vi "Test bearbeiten.vi"(6 "error in (no error)":errorcluster, 8 "Test in":refnum<class "Test.lvclass">, 9 "Data":T1={"Report.lvclass"=refnum, "Norm"="", "last State"=enum."Initialize", "Norm ID"=0, "parameter"=[], "EMTestCWS500N.lvclass"=refnum, "CEG4500.lvclass"=refnum, "Tektronix RSA5106A.lvclass"=refnum, "erfolgreich"=FALSE, "log"="", "Kommentar"="", "Device Enum"=enum."emTestCWS500N", "Test Enum"=enum."HF-Felder", "debug"=FALSE, "tab"=enum."Hauptmenü", "ESD Pistol.lvclass"=refnum, "SubPnl Refnum"=refnum, "TabCtl Refnum"=refnum, "ButtonsEinblenden?"=FALSE, "VKey"=enum."ASCII"}) -> (0 "error out":errorcluster, 1 "abbrechen":bool, 2 "Test out":refnum<class "Test.lvclass">)   [LabVIEW 2013, in "DataCreation.lvlib"]
uses:
  lib/DataCreation.lvlib
  Main/controls/Data.ctl
  classes/Datastructure/Report/Report.lvclass
  classes/Devices/emTestCWS500N/EMTestCWS500N.lvclass
  classes/Devices/CEG4500/CEG4500.lvclass
  classes/Devices/Tektronix RSA5106A/Tektronix RSA5106A.lvclass
  ESD Pistol.lvclass
  Main/controls/State.ctl
  classes/Devices/DeviceInterface/Devices.ctl
  classes/Tests/TestInterface/Tests.ctl
  Tabs.ctl
  <vilib>/event_ctls.llb/eventvkey.ctl
  classes/Datastructure/Test/Test.lvclass
  classes/Datastructure/Image/img.lvclass
  classes/Datastructure/Norm/Norm.lvclass
  lib/TreeRepresentation.lvlib
panel:
  in  "number of pictures":i32
  in  "Tab Control":enum32{"Test", "Daten"}(tab)
  in  "Cancel Button":bool
  in  "Tree pics":string(tree)
  in  "OK Button":bool
  in  "Add picture":bool
  in  "Kommentar":string
  in  "Test Name":string
  in  "Parameter":string[][](table)
  in  "Tree Report":string(tree)
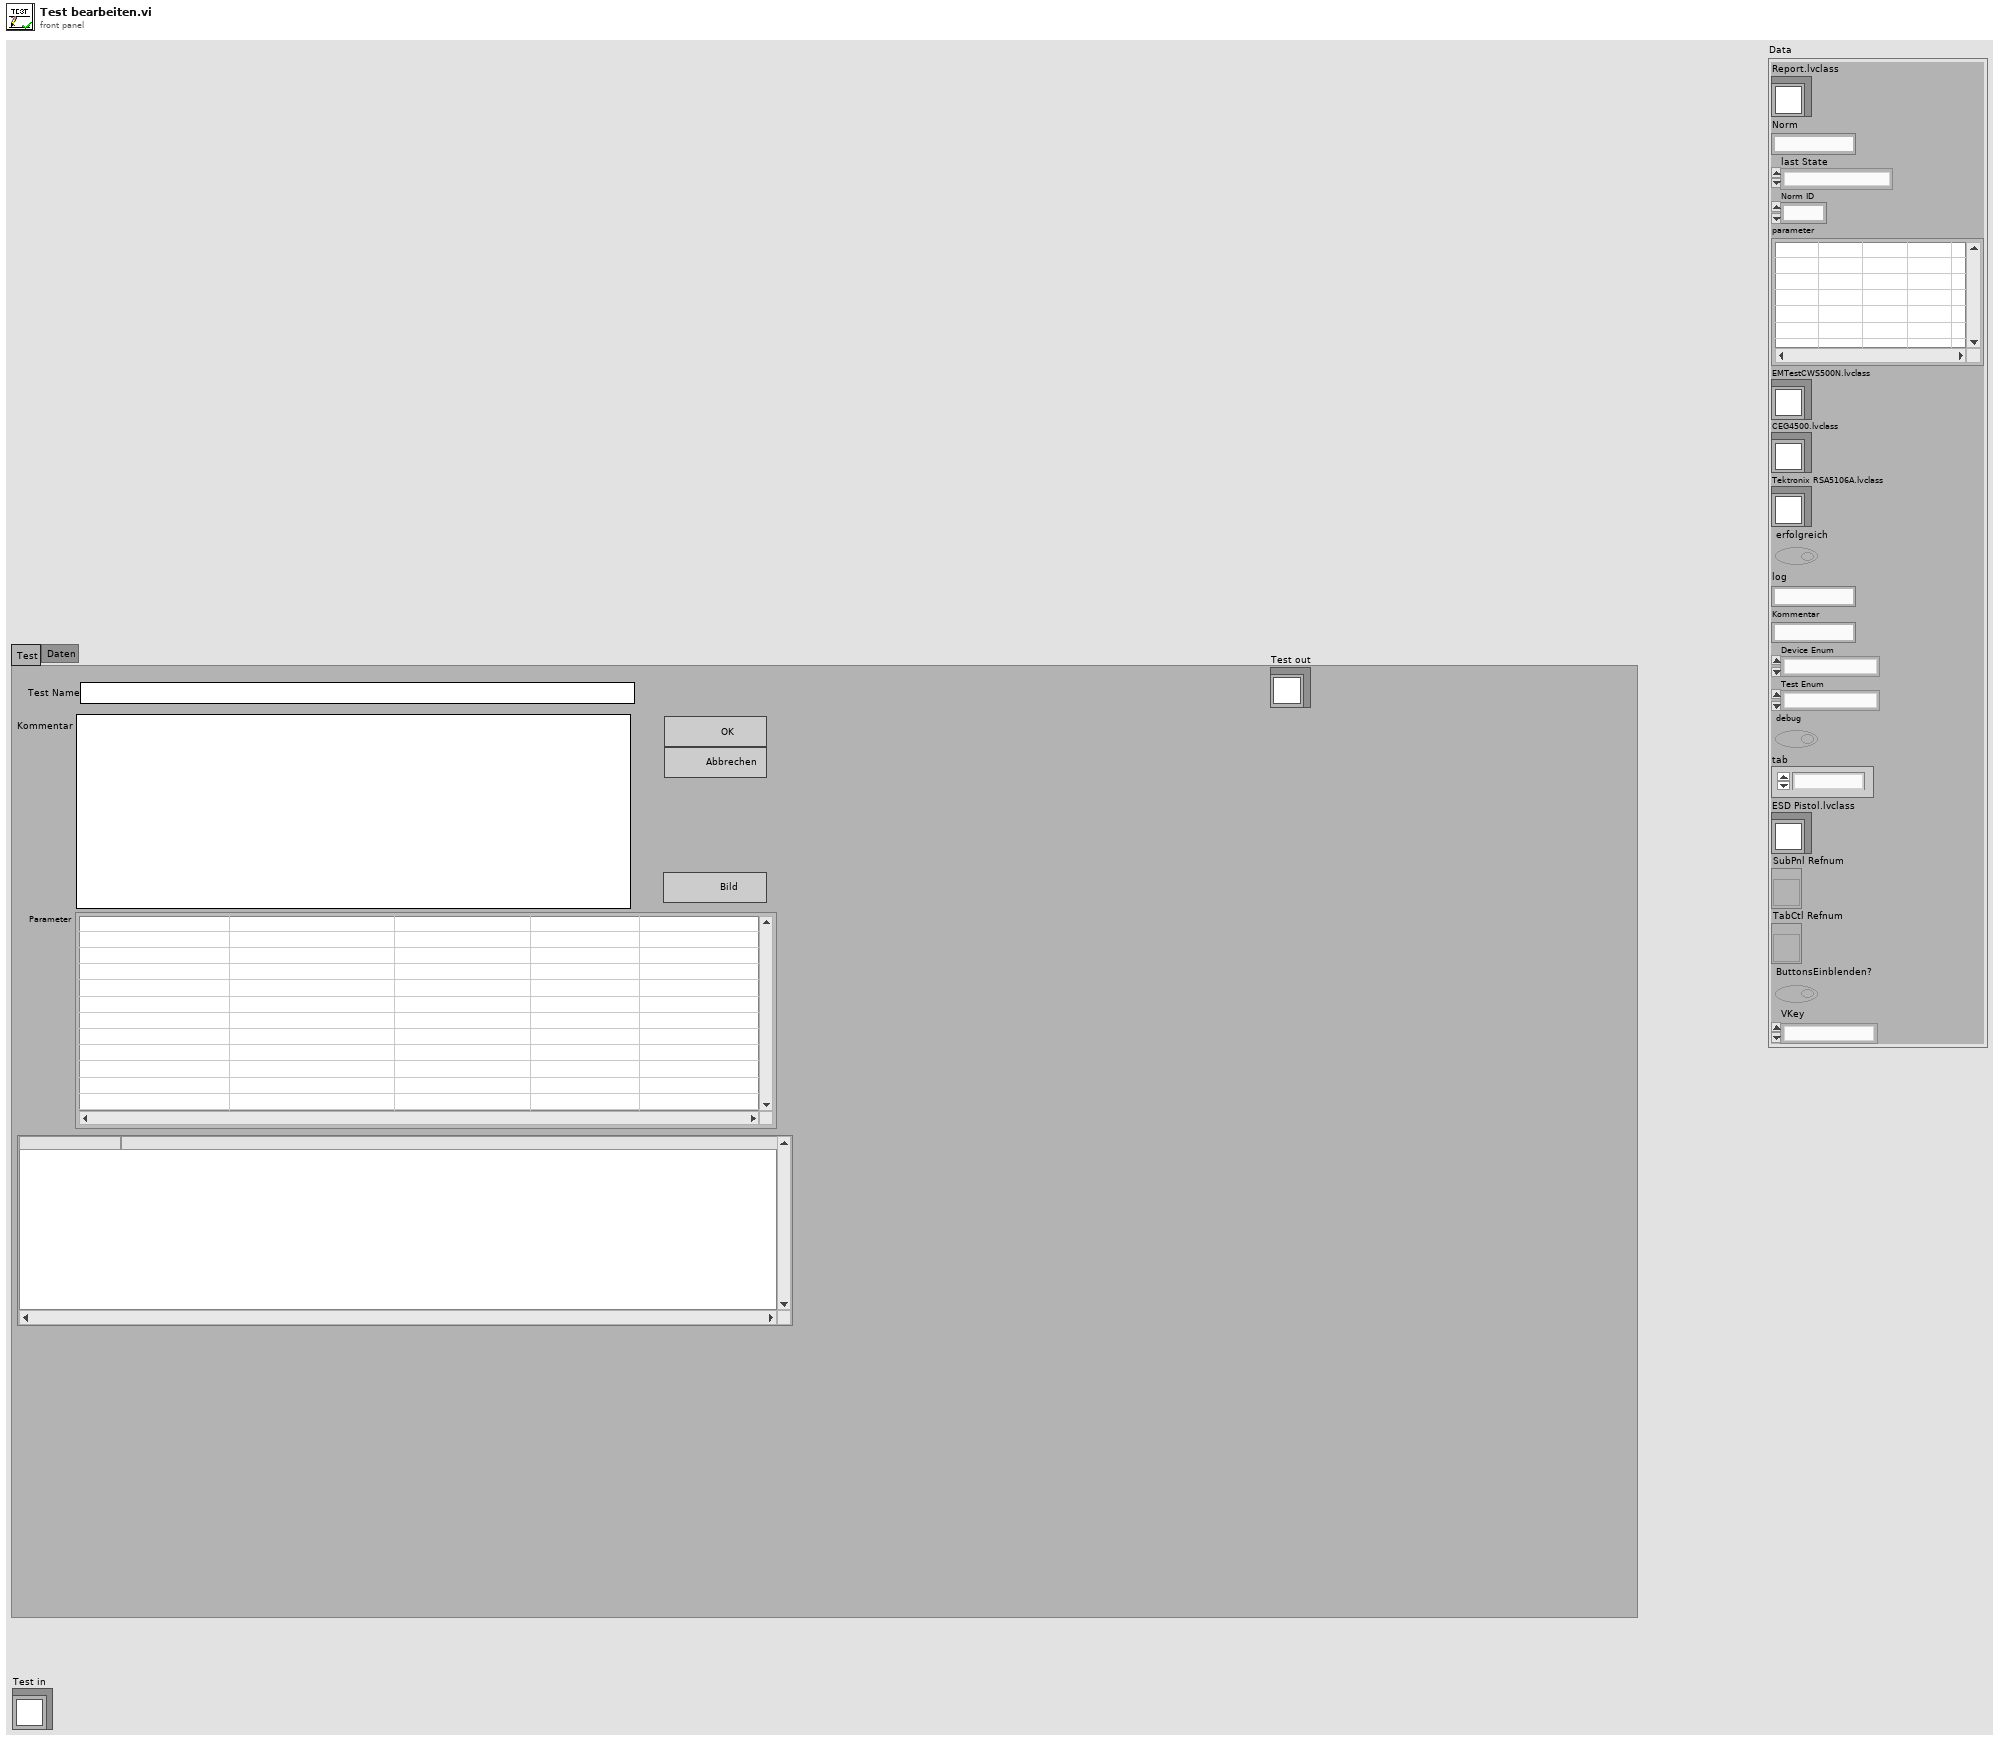
[diagram p1: front panel]
types:
  T1 = typedef "Data.ctl" = cluster{"Report.lvclass":refnum<class "Report.lvclass">, "Norm":string, "last State":T2, "Norm ID":i32, "parameter":string[][], "EMTestCWS500N.lvclass":refnum<class "EMTestCWS500N.lvclass">, "CEG4500.lvclass":refnum<class "CEG4500.lvclass">, "Tektronix RSA5106A.lvclass":refnum<class "Tektronix RSA5106A.lvclass">, "erfolgreich":bool, "log":string, "Kommentar":string, "Device Enum":T3, "Test Enum":T4, "debug":bool, "tab":T5, "ESD Pistol.lvclass":refnum<class "ESD Pistol.lvclass">, "SubPnl Refnum":refnum<vi>, "TabCtl Refnum":refnum<vi>, "ButtonsEinblenden?":bool, "VKey":T6}
  T2 = typedef "State.ctl" = enum16{"create Pdf", "edit Report", "load Report", "save Report", "do Test", "CDN Kalibrierung", "enter Report Parameters", "new Test", "Protokoll", "read Tree", "update Tree", "Fehler", "Initialize", "Wait for Event", "Exit"}
  T3 = typedef "Devices.ctl" = enum16{"unbekannt", "ESD Pistol", "Tektronix RSA5106A", "emTestCWS500N", "CEG-4500"}
  T4 = typedef "Tests.ctl" = enum16{"unbekannt", "Störaussendung", "Burst", "ESD", "Surge", "Spannungseinbruch", "HF-Felder"}
  T5 = typedef "Tabs.ctl" = enum32{"Hauptmenü", "Prüfbericht", "Einstellungen"}
  T6 = typedef "eventvkey.ctl" = enum16{"ASCII", "Enter", "Return", "Shift", "Ctrl", "Alt", "Cmd", "Opt", "Caps", "NumLock", "Clear", "Break", "Up", "Down", "Left", "Right", "Insert", "Delete", "Home", "End", "PageUp", "PageDown", "Escape", "Help", "Pause", "ScrollLock", "F1", "F2", "F3", "F4", "F5", "F6", "F7", "F8", "F9", "F10", "F11", "F12", "F13", "F14", "F15", "F16", "F17", "F18", "F19", "F20", "F21", "F22", "F23", "F24", "Play", "VolumeUp", "VolumeDown", "Mute", "Two Byte Char"}
  T7 = enum16{"abbrechen", "create obj", "add pic", "init", "wait for event"}
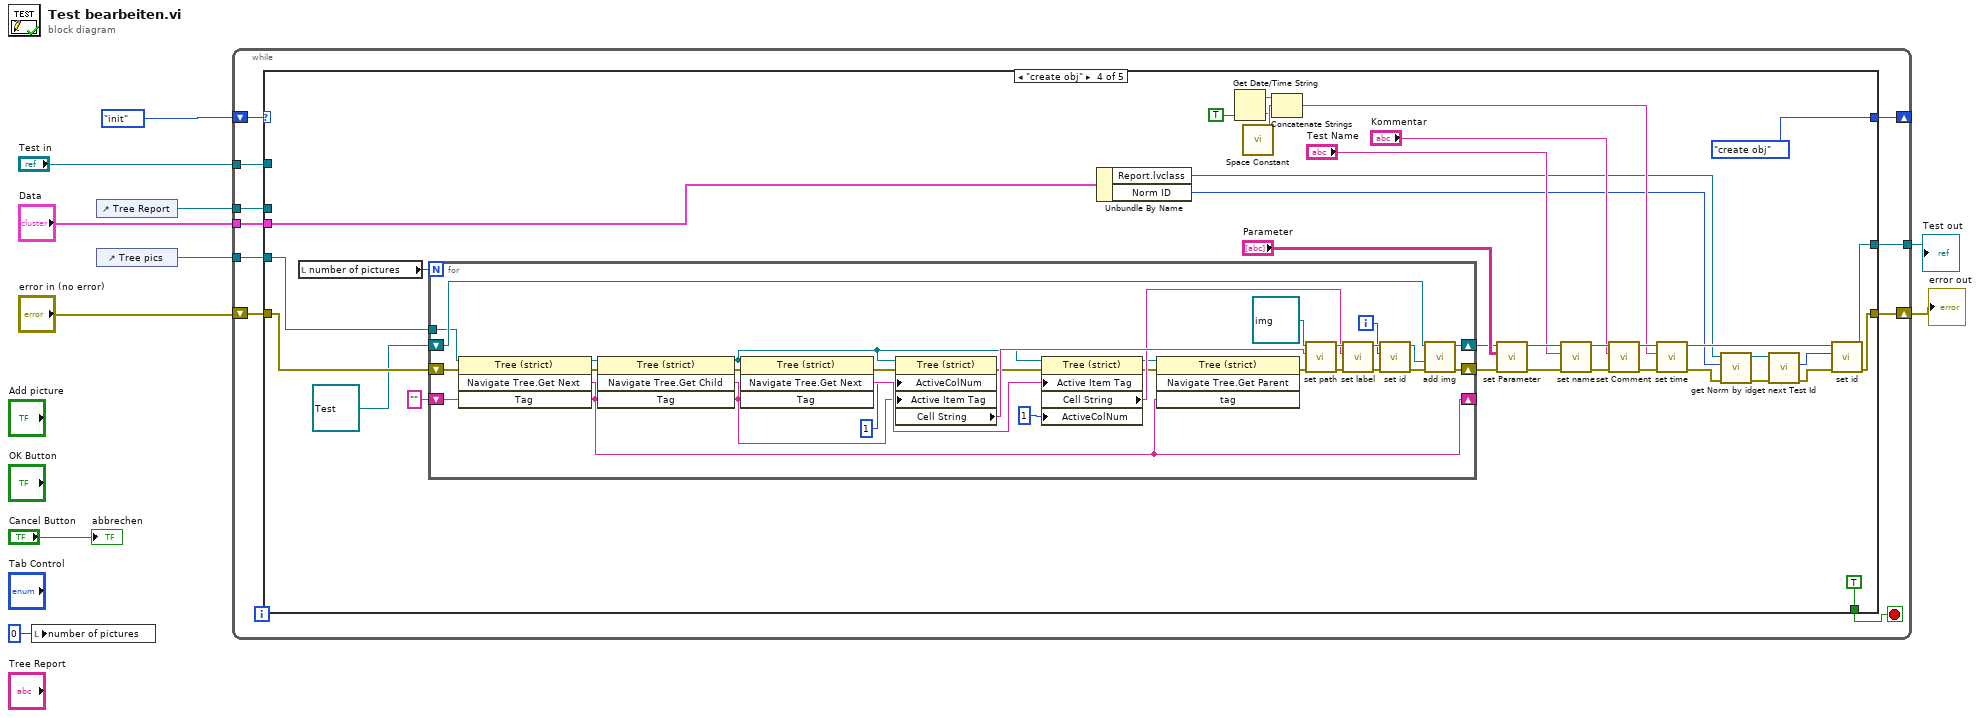
[diagram p0: block diagram]
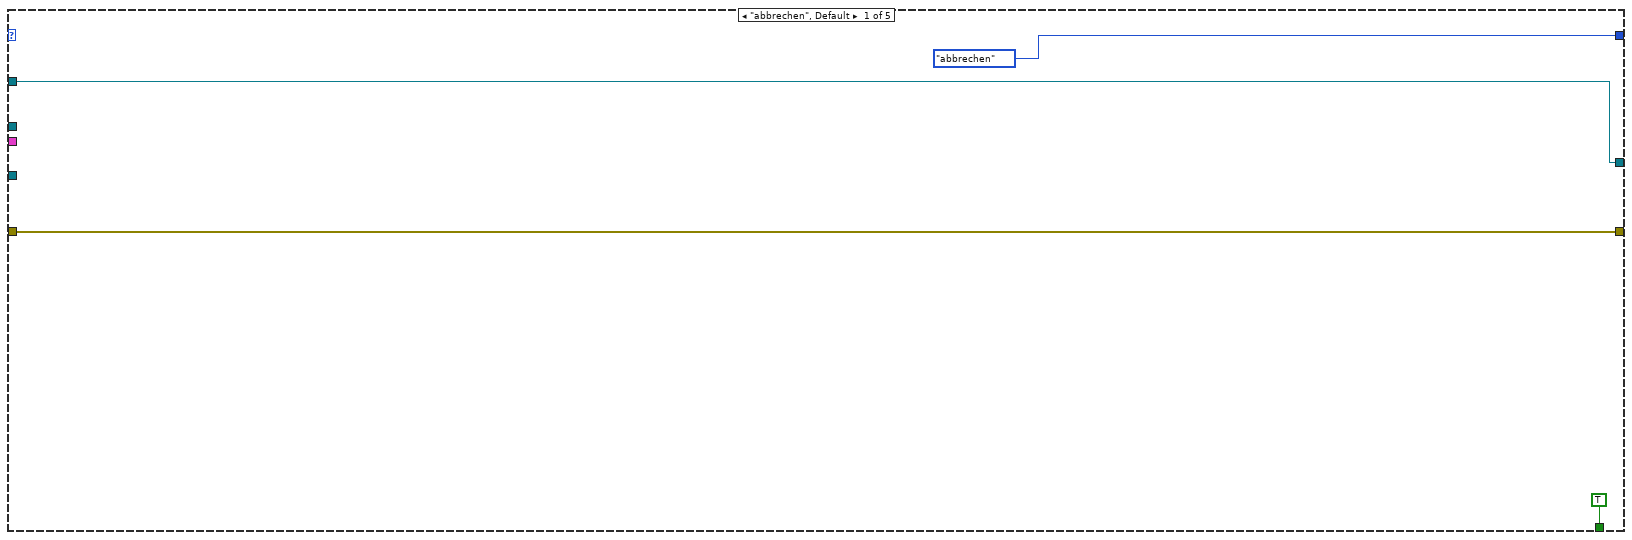
[diagram p2: hidden frame]
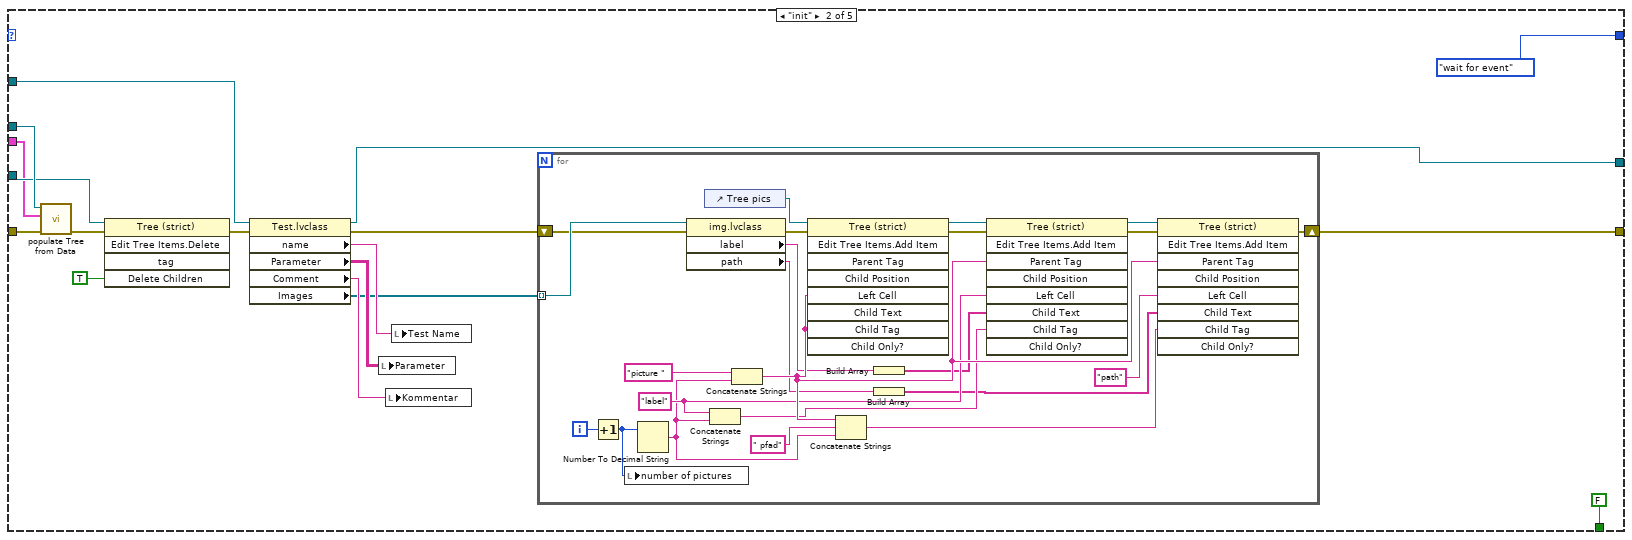
[diagram p3: hidden frame]
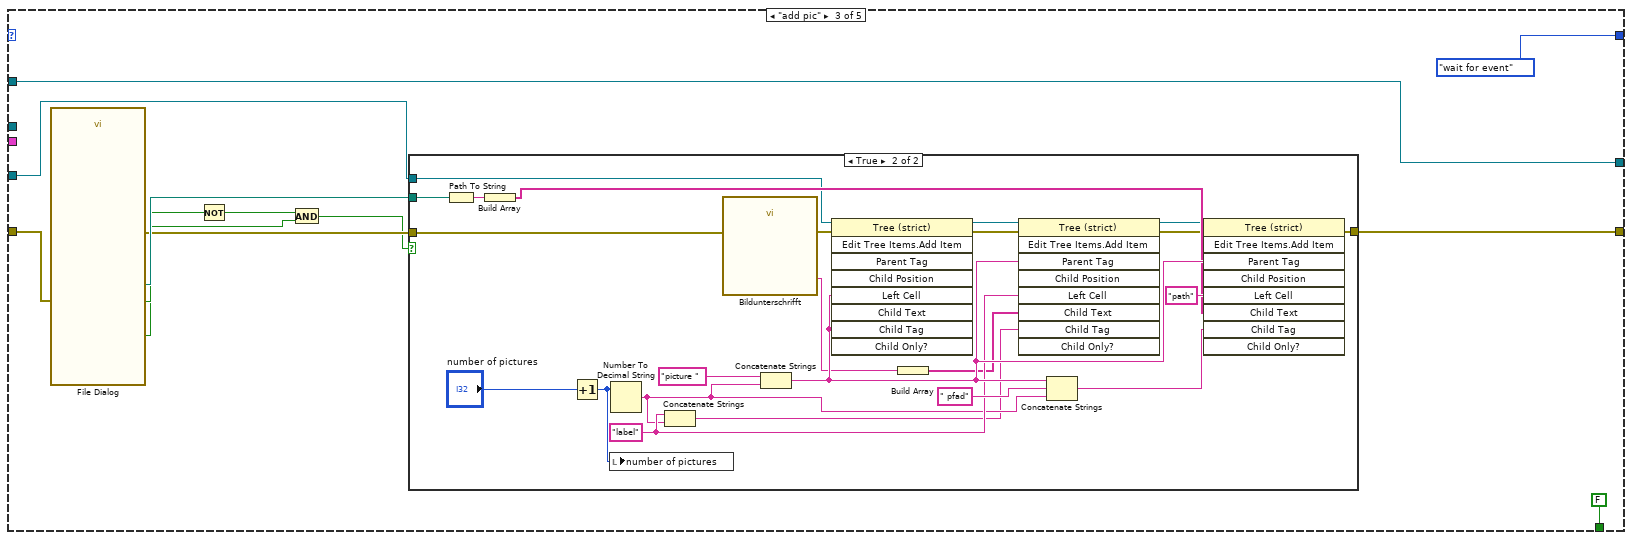
[diagram p4: hidden frame]
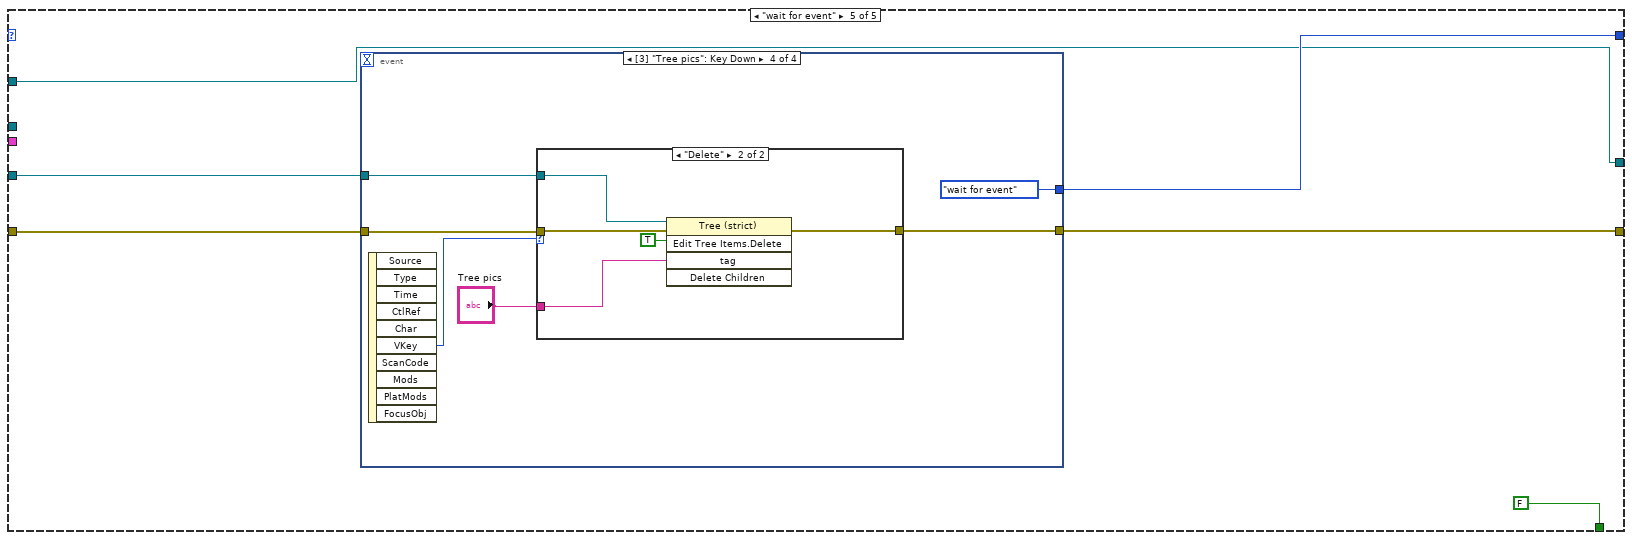
[diagram p6: hidden frame]
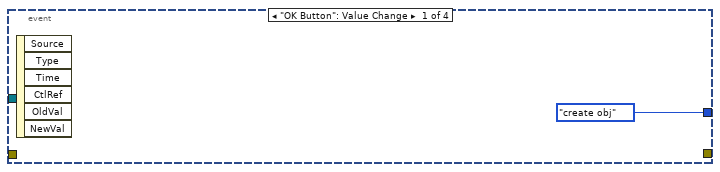
[diagram p7: hidden frame]
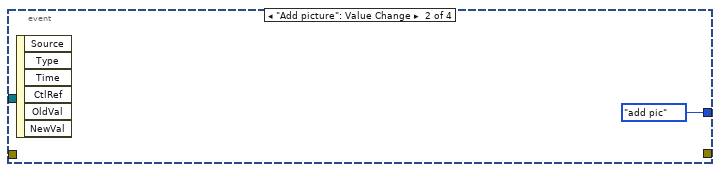
[diagram p8: hidden frame]
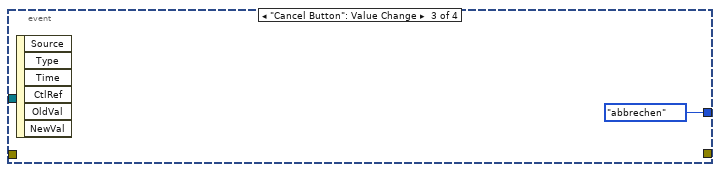
[diagram p9: hidden frame]
diagram:
  n1 = local write "number of pictures"(0 ("number of pictures")) -> ()
  n2 = control-ref of="Tree Report"() -> (w10:refnum<vi>)
  n3 = control-ref of="Tree pics"() -> (w8:refnum<vi>)
  n4 = while {
    tunnel: w10 -> [w20]
    tunnel: w8 -> [w18]
    tunnel: "Data" -> [w17]
    tunnel: "Test in" -> [w15]
    tunnel: [w14] -> w1
    shift-right: [w12] -> _
    shift-left: T7."init" -> [w13]
    shift-right: [w16] -> w2
    shift-left: "error in (no error)" -> [w19]
    stop <- w11 stop-if-true
    n5 = case shown="\"create obj\"" w13 {
      tunnel: w20 -> [_ w41 _ _ _]
      tunnel: w19 -> [w23 w40 w70 w117 w167]
      tunnel: w18 -> [_ w39 w68 w116 w169]
      tunnel: w17 -> [_ w37 _ w108 _]
      tunnel: [w23 w31 w69 w112 w168] -> w16
      tunnel: w15 -> [w24 w30 w66 _ w166]
      tunnel: [w24 w27 w66 w111 w166] -> w14
      tunnel: [T7."abbrechen" T7."wait for event" T7."wait for event" T7."create obj" w170] -> w12
      tunnel: [TRUE FALSE FALSE TRUE FALSE] -> w11
      frame "abbrechen", Default {
      }
      frame "init" {
        n6 = call "populate Tree from Data.vi"("error in (no error)"=w40, "Data"=w37, "reference"=w41) -> ("error out"=w33:errorcluster)  [unwired: 6 in]
        n7 = invoke class="Tree (strict)" method="Edit Tree Items.Delete"(reference=w39, error in=w33, "Delete Children"=TRUE ("Unterobjekte löschen?")) -> (error out=w29:errorcluster)  [unwired: 2 in, 4 out]
        n8 = property class="Test.lvclass"(reference=w30, error in=w29) -> (reference out=w27:refnum<class "Test.lvclass">, error out=w28:errorcluster, "name"=w34:string, "Parameter"=w36:string[][], "Comment"=w35:string, "Images"=w32:refnum<class "img.lvclass">[])
        n9 = local write "Parameter"(w36) -> ()
        n10 = local write "Kommentar"(w35) -> ()
        n11 = local write "Test Name"(w34) -> ()
        n12 = for {
          tunnel: w32 -> [w48] mode=indexing
          shift-right: [w43] -> w31
          shift-left: w28 -> [w47]
          i -> [w49]
          w58 = "label" ("Left Cell String")
          n13 = Increment(x=w49) -> (x+1=w42:i32)
          n14 = local write "number of pictures"(w42) -> ()
          n15 = Number To Decimal String(number=w42) -> (decimal integer string=w57:string)  [unwired: 1 in]
          n16 = property class="img.lvclass"(reference=w48, error in=w47) -> (error out=w46:errorcluster, "label"=w45:string, "path"=w44:string)  [unwired: 1 out]
          n17 = control-ref of="Tree pics"() -> (w64:refnum<vi>)
          n18 = Concatenate Strings(w58, w57) -> (w56:string)
          n19 = Concatenate Strings("picture " ("Left Cell String"), w57) -> (w59:string)
          n20 = invoke class="Tree (strict)" method="Edit Tree Items.Add Item"(reference=w64, error in=w46, "Left Cell"=w59, "Child Tag"=w59) -> (reference out=w54:refnum<vi>, error out=w51:errorcluster)  [unwired: 5 in, 7 out]
          n21 = Concatenate Strings(w59, " pfad", w57) -> (w61:string)
          n22 = Build Array(w45) -> (w52:string[])
          n23 = Build Array(w44) -> (w55:string[])
          n24 = invoke class="Tree (strict)" method="Edit Tree Items.Add Item"(reference=w54, error in=w51, "Parent Tag"=w59, "Left Cell"=w58, "Child Text"=w52, "Child Tag"=w56) -> (reference out=w53:refnum<vi>, error out=w50:errorcluster)  [unwired: 3 in, 7 out]
          n25 = invoke class="Tree (strict)" method="Edit Tree Items.Add Item"(reference=w53, error in=w50, "Parent Tag"=w59, "Left Cell"="path" ("Left Cell String"), "Child Text"=w55, "Child Tag"=w61) -> (error out=w43:errorcluster)  [unwired: 3 in, 8 out]
        }
      }
      frame "add pic" {
        n26 = call "File Dialog"("error in"=w70) -> ("selected path"=w76:path, "exists"=w71:bool, "cancelled"=w74:bool, "error out"=w75:errorcluster)  [unwired: 11 in]
        n27 = Not(x=w74) -> (.not. x?=w72:bool)
        n28 = And(x=w72, y=w71) -> (x .and. y?=w73:bool)
        n29 = case shown="True" w73 {
          tunnel: w76 -> [_ w92]
          tunnel: w75 -> [w77 w87]
          tunnel: [w77 w79] -> w69
          tunnel: w68 -> [_ w78]
          frame False {
          }
          frame True {
            w95 = "label" ("Left Cell String")
            n30 = Path To String(path=w92) -> (string=w88:string)
            n31 = Build Array(w88) -> (w91:string[])
            n32 = Increment(x="number of pictures") -> (x+1=w83:i32)
            n33 = local write "number of pictures"(w83) -> ()
            n34 = Number To Decimal String(number=w83) -> (decimal integer string=w94:string)  [unwired: 1 in]
            n35 = Concatenate Strings(w95, w94) -> (w93:string)
            n36 = call "Bildunterschrifft"("error in (no error)"=w87) -> ("Bildunterschrifft"=w86:string, "error out"=w82:errorcluster)  [unwired: 16 in, 1 out]
            n37 = Concatenate Strings("picture " ("Left Cell String"), w94) -> (w96:string)
            n38 = invoke class="Tree (strict)" method="Edit Tree Items.Add Item"(reference=w78, error in=w82, "Left Cell"=w96, "Child Tag"=w96) -> (reference out=w90:refnum<vi>, error out=w81:errorcluster)  [unwired: 5 in, 7 out]
            n39 = Build Array(w86) -> (w85:string[])
            n40 = invoke class="Tree (strict)" method="Edit Tree Items.Add Item"(reference=w90, error in=w81, "Parent Tag"=w96, "Left Cell"=w95, "Child Text"=w85, "Child Tag"=w93) -> (reference out=w89:refnum<vi>, error out=w80:errorcluster)  [unwired: 3 in, 7 out]
            n41 = Concatenate Strings(w96, " pfad", w94) -> (w98:string)
            n42 = invoke class="Tree (strict)" method="Edit Tree Items.Add Item"(reference=w89, error in=w80, "Parent Tag"=w96, "Left Cell"="path" ("Left Cell String"), "Child Text"=w91, "Child Tag"=w98) -> (error out=w79:errorcluster)  [unwired: 3 in, 8 out]
          }
        }
      }
      frame "create obj" {
        n43 = local read "number of pictures"() -> (w115:i32)
        n44 = for {
          N: w115 -> [_]
          tunnel: w116 -> [w145]
          shift-right: [w156] -> w129
          shift-left: refnum<class "Test.lvclass"> refnum ("Test (Ausgang)") -> [w163]
          shift-right: [w150] -> w130
          shift-left: w117 -> [w149]
          shift-right: [w144] -> _
          shift-left: "" ("Navigate Tree:Get Next Item") -> [w143]
          i -> [w137]
          n45 = invoke class="Tree (strict)" method="Navigate Tree.Get Next"(reference=w145, error in=w149, "Tag"=w143) -> (reference out=w164:refnum<vi>, error out=w155:errorcluster, "Navigate Tree:Get Next Item"=w144:string)  [unwired: 1 in, 1 out]
          n46 = invoke class="Tree (strict)" method="Navigate Tree.Get Child"(reference=w164, error in=w155, "Tag"=w144) -> (reference out=w159:refnum<vi>, error out=w154:errorcluster, "Navigate Tree:Get Child"=w142:string)  [unwired: 1 in, 1 out]
          n47 = invoke class="Tree (strict)" method="Navigate Tree.Get Next"(reference=w159, error in=w154, "Tag"=w142) -> (error out=w153:errorcluster, "Navigate Tree:Get Next Item"=w158:string)  [unwired: 1 in, 2 out]
          n48 = property class="Tree (strict)"(reference=w159, error in=w153, "ActiveColNum"=1 ("Active Cell:Active Column Number"), "Active Item Tag"=w142) -> (error out=w152:errorcluster, "Cell String"=w160:string)  [unwired: 1 out]
          n49 = property class="Tree (strict)"(reference=w159, error in=w152, "Active Item Tag"=w158, "ActiveColNum"=1 ("Active Cell:Active Column Number")) -> (reference out=w146:refnum<vi>, error out=w141:errorcluster, "Cell String"=w157:string)
          n50 = invoke class="Tree (strict)" method="Navigate Tree.Get Parent"(reference=w146, error in=w141, "tag"=w144) -> (error out=w140:errorcluster)  [unwired: 1 in, 3 out]
          n51 = call-dynamic "set path.vi"("error in (no error)"=w140, "path"=w160, "img (Eingang)"=refnum<class "img.lvclass"> refnum ("img.lvclass")) -> ("error out"=w151:errorcluster, "img (Ausgang)"=w162:refnum<class "img.lvclass">)  [unwired: 7 in]
          n52 = call-dynamic "set label.vi"("error in (no error)"=w151, "label"=w157, "img (Eingang)"=w162) -> ("error out"=w139:errorcluster, "img (Ausgang)"=w138:refnum<class "img.lvclass">)  [unwired: 7 in]
          n53 = call-dynamic "set id.vi"("error in (no error)"=w139, "id"=w137, "img in"=w138) -> ("error out"=w136:errorcluster, "img out"=w135:refnum<class "img.lvclass">)  [unwired: 7 in]
          n54 = call-dynamic "add img.vi"("error in (no error)"=w136, "img.lvclass"=w135, "Test (Eingang)"=w163) -> ("error out"=w150:errorcluster, "Test (Ausgang)"=w156:refnum<class "Test.lvclass">)  [unwired: 6 in]
        }
        n55 = Unbundle By Name(w108) -> ("Report.lvclass"=w106:refnum<class "Report.lvclass">, "Norm ID"=w105:i32)
        n56 = Get Date/Time String(want seconds? (F)=TRUE) -> (date string=w121:string, time string=w120:string)  [unwired: 2 out]
        n57 = call <vilib>:"Space Constant.vi"() -> ("String"=w122:string)
        n58 = Concatenate Strings(w121, w122, w120) -> (w124:string)
        n59 = call-dynamic "set Parameter.vi"("error in (no error)"=w130, "Parameter"="Parameter", "Test (Eingang)"=w129) -> ("error out"=w133:errorcluster, "Test (Ausgang)"=w132:refnum<class "Test.lvclass">)  [unwired: 7 in]
        n60 = call-dynamic "set name.vi"("error in (no error)"=w133, "name"="Test Name", "Test (Eingang)"=w132) -> ("error out"=w128:errorcluster, "Test (Ausgang)"=w125:refnum<class "Test.lvclass">)  [unwired: 7 in]
        n61 = call-dynamic "set Comment.vi"("error in (no error)"=w128, "Comment"="Kommentar", "Test (Eingang)"=w125) -> ("error out"=w127:errorcluster, "Test (Ausgang)"=w126:refnum<class "Test.lvclass">)  [unwired: 7 in]
        n62 = call-dynamic "set time.vi"("error in (no error)"=w127, "time"=w124, "Test (Eingang)"=w126) -> ("error out"=w104:errorcluster, "Test (Ausgang)"=w134:refnum<class "Test.lvclass">)  [unwired: 7 in]
        n63 = call-dynamic "get Norm by id.vi"("error in (no error)"=w104, "id"=w105, "Report (Eingang)"=w106) -> ("error out"=w103:errorcluster, "Norm.lvclass"=w107:refnum<class "Norm.lvclass">)  [unwired: 4 in, 3 out]
        n64 = call-dynamic "get next Test Id.vi"("error in (no error)"=w103, "Norm in"=w107) -> ("error out"=w101:errorcluster, "id"=w102:u32)  [unwired: 7 in, 1 out]
        n65 = call-dynamic "set id.vi"("error in (no error)"=w101, "id"=w102, "Test in"=w134) -> ("error out"=w112:errorcluster, "Test out"=w111:refnum<class "Test.lvclass">)  [unwired: 7 in]
      }
      frame "wait for event" {
        n66 = event shown="[3] \"Tree pics\": Key Down" {
          selector: _ -> [_ _ _ _]
          dyn-events: _ -> [_ _ _ _]
          timeout: _ -> [_ _ _ _]
          tunnel: [T7."create obj" T7."add pic" T7."abbrechen" T7."wait for event"] -> w170
          tunnel: w169 -> [_ _ _ w178]
          tunnel: [_ _ _ w177] -> w168
          tunnel: w167 -> [_ _ _ w176]
          event "OK Button": Value Change {
            n67 = event-data() -> ()  [unwired: 1 in, 6 out]
          }
          event "Add picture": Value Change {
            n68 = event-data() -> ()  [unwired: 1 in, 6 out]
          }
          event "Cancel Button": Value Change {
            n69 = event-data() -> ()  [unwired: 1 in, 6 out]
          }
          event "Tree pics": Key Down {
            n70 = event-data() -> ("VKey"=w174:T6)  [unwired: 1 in, 9 out]
            n71 = case shown="\"Delete\"" w174 {
              tunnel: "Tree pics" -> [_ w183]
              tunnel: w178 -> [_ w184]
              tunnel: [w180 w182] -> w177
              tunnel: w176 -> [w180 w181]
              frame "ASCII", Default {
              }
              frame "Delete" {
                n72 = invoke class="Tree (strict)" method="Edit Tree Items.Delete"(reference=w184, error in=w181, "tag"=w183, "Delete Children"=TRUE ("Delete Children?")) -> (error out=w182:errorcluster)  [unwired: 1 in, 4 out]
              }
            }
          }
        }
      }
    }
  }
  "error out" <- w2
  "Test out" <- w1
  "abbrechen" <- "Cancel Button"
